vi "Set Serial Interface Max Baud.vi"(8 "Error In":errorcluster, 10 "Baud Rate":T1, 11 "LINX Device Config":T2) -> (0 "Error Out":errorcluster, 3 "LINX Device Config":T2)   [LabVIEW 2011, in "LMH-LINX.lvlib" / "Device.lvlib"]
doc: "Set the maximum baud rate the LINX device is capable of using to communicate with the host."
uses:
  Device.lvlib
  Type Defs/LINX Device Config.ctl
  Type Defs/Interface.ctl
  Type Defs/TCP Config.ctl
  Type Defs/Channels.ctl
  Type Defs/Baud Rate.ctl
  Type Defs/Error Type.ctl
  LMH-LINX.lvlib
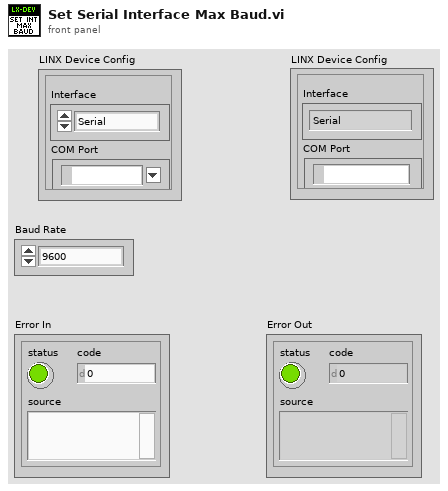
[diagram p1: front panel]
types:
  T1 = typedef "LMH-LINX.lvlib/Baud Rate.ctl" = enum16{"9600", "14400", "19200", "28800", "38400", "57600", "115200"}
  T2 = typedef "LMH-LINX.lvlib/Device.lvlib/LINX Device Config.ctl" = cluster{"Interface":T3, "COM Port":refnum<visa-resource-name>, "TCP Configuration":T4, "Device Family":u8, "Device ID":u8, "Device Name":string, "TCP Ref":refnum<k5>, "Channels":T5}
  T3 = typedef "LMH-LINX.lvlib/Interface.ctl" = enum16{"Serial", "TCP"}
  T4 = typedef "LMH-LINX.lvlib/Device.lvlib/TCP Config.ctl" = cluster{"IP Address":string, "Port":u16}
  T5 = typedef "LMH-LINX.lvlib/Channels.ctl" = cluster{"DI":u8[], "DO":u8[], "AI":u8[], "AO":u8[], "PWM":u8[], "QE":u8[], "UART":u8[], "I2C 2":u8[], "SPI":u8[], "CAN":u8[], "Servo":u8[], "AI Ref (V)":dbl, "AO Ref (V)":dbl, "AO Resolution (Bits)":u8}
  T6 = typedef "LMH-LINX.lvlib/Error Type.ctl" = enum16{"Unknown", "Timeout", "Corrupt Return Packet", "Unable To Connect", "Command Not Supported", "Channel DNE", "Invalid COM Config", "Firmware Version Mismatch", "myRIO Support", "CMD Specific Error"}
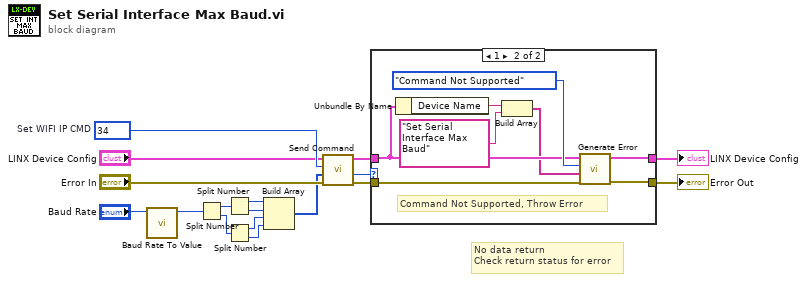
[diagram p0: block diagram]
diagram:
  w16 = u16 34  # Set WIFI IP CMD
  # "No data return\nCheck return status for error"
  n1 = call "Baud Rate To Value.vi"("Baud Rate"="Baud Rate") -> ("Baud Rate Value"=w1:u32)  [unwired: 10 in]
  n2 = Split Number(x=w1) -> (hi(x)=w9:u16, lo(x)=w8:u16)
  n3 = Split Number(x=w9) -> (hi(x)=w7:u8, lo(x)=w6:u8)
  n4 = Split Number(x=w8) -> (hi(x)=w4:u8, lo(x)=w5:u8)
  n5 = Build Array(w7, w6, w4, w5) -> (w10:u8[])
  n6 = call "Send Command.vi"("Error In"="Error In", "ARGS"=w10, "CMD"=w16, "LINX Device Config"="LINX Device Config") -> ("Error Out"=w11:errorcluster, "Status"=w3:u8, "LINX Device Config"=w13:T2)  [unwired: 4 in, 1 out]
  n7 = case shown="1" w3 {
    tunnel: [w18 w25] -> w14
    tunnel: w13 -> [w18 w21]
    tunnel: [w19 w26] -> w12
    tunnel: w11 -> [w19 w27]
    frame 0, Default {
      # "Status OK, Process Data"
    }
    frame 1 {
      # "Command Not Supported, Throw Error"
      n8 = Unbundle By Name(w21) -> ("Device Name"=w22:string)
      n9 = Build Array(w22, "Set Serial Interface Max Baud") -> (w20:string[])
      n10 = call "Generate Error.vi"("Error In"=w27, "Arguments"=w20, "Error Type"=Error_Type."Command Not Supported", "LINX Device Config"=w21) -> ("Error Out"=w26:errorcluster, "LINX Device Config"=w25:T2)  [unwired: 6 in]
    }
  }
  "Error Out" <- w12
  "LINX Device Config" <- w14
